vi "Simple Endpoint Control.vi"(3 "error in":errorcluster, 4 "Side":T1=enum."right", 5 "Position":T2={"Theta"=-42.91139240506329, "r"=17.78481012658228, "wrist"=-20.886075949367083, "Z"=0.25316455696202533} {"Z" scale=-10.0..10.0; "wrist" scale=-90.0..90.0; "r" scale=10.0..25.0; "Theta" scale=-90.0..90.0}) -> (0 "error out":errorcluster)   [LabVIEW 2010]
uses:
  <userlib>/ROSforLV_0.1/ROS/Code/SubVIs/BaxterArmsSmall.ctl
  <userlib>/ROSforLV_0.1/ROS/Code/SubVIs/BaxterSide.ctl
panel:
  out "g":dbl=49.666540029773564
  out "x":dbl=17.786611918279583
  out "p":dbl=0.8155432028971262
  out "a":dbl=54.75975470538772
  in  "Start":T3={"Elbow 0"=0.0, "Elbow 1"=55.8123726628928, "Shoulder 0"=0.0, "Shoulder 1"=-28.952431226064945, "Wrist 0"=0.0, "Wrist 1"=63.14005856317215, "Wrist 2"=0.0}
  out "Arm Angles (degrees)":T3={"Elbow 0"=0.0, "Elbow 1"=104.42629473516128, "Shoulder 0"=-42.91139240506329, "Shoulder 1"=-55.575297908284846, "Wrist 0"=0.0, "Wrist 1"=41.14900317312356, "Wrist 2"=-20.886075949367083}
  in  "d 4":dbl=10.0
  in  "d 3":dbl=15.0
  in  "d 2":dbl=14.0
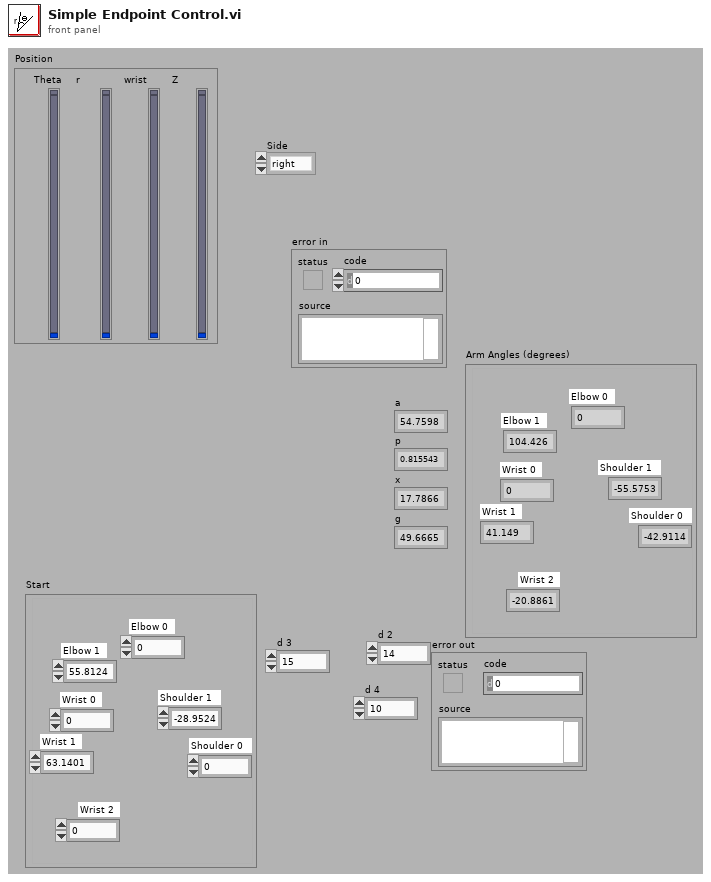
[diagram p1: front panel]
types:
  T1 = typedef "BaxterSide.ctl" = enum16{"left", "right"}
  T2 = cluster{"Theta":dbl, "r":dbl, "wrist":dbl, "Z":dbl}
  T3 = typedef "BaxterArmsSmall.ctl" = cluster{"Elbow 0":dbl, "Elbow 1":dbl, "Shoulder 0":dbl, "Shoulder 1":dbl, "Wrist 0":dbl, "Wrist 1":dbl, "Wrist 2":dbl}
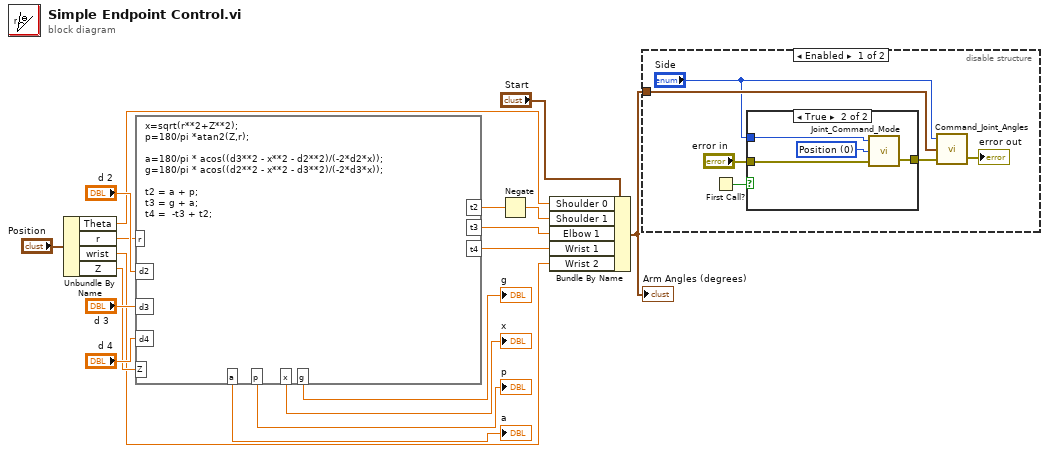
[diagram p0: block diagram]
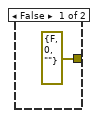
[diagram p2: hidden frame]
diagram:
  n1 = Unbundle By Name("Position") -> ("Theta"=w4:dbl, "r"=w3:dbl, "wrist"=w1:dbl, "Z"=w2:dbl)
  n2 = formula code="x=sqrt(r**2+Z**2);\np=180/pi *atan2(Z,r);\n\na=180/pi * acos((d3**2 - x**2 - d2**2)/(-2*d2*x));\ng=180/pi * acos((d2**2 - x**2 - d3**2)/(-2*d3*x));\n\nt2 = a + p;\nt3 = g + a;\nt4 =  -t3 + t2;"("r"=w3, "d2"="d 2", "d3"="d 3", "d4"="d 4", "Z"=w2) -> ("t2"=w13:dbl, "t3"=w12:dbl, "t4"=w11:dbl, "a"=→"a":dbl, "p"=→"p":dbl, "x"=→"x":dbl, "g"=→"g":dbl)
  n3 = Negate(x=w13) -> (-x=w6:dbl)
  n4 = Bundle By Name(cluster="Start", "Shoulder 0"=w4, "Shoulder 1"=w6, "Elbow 1"=w12, "Wrist 1"=w11, "Wrist 2"=w1) -> (w17:T3)
  "Arm Angles (degrees)" <- w17
  n5 = disable-structure shown="Enabled" {
    disable-tunnel: w17 -> [w24 _]
    frame Enabled {
      n6 = First Call?() -> (First Call?: T/F=w22:bool)
      n7 = case shown="True" w22 {
        tunnel: [errorcluster {"status"=FALSE, "code"=0, "source"=""} ("error out") w28] -> w23
        tunnel: "Side" -> [_ w27]
        tunnel: "error in" -> [_ w26]
        frame False {
        }
        frame True {
          w29 = u8 0 items=["Position", "Velocity", "Effort"] ("Mode")
          n8 = call <userlib>:"Joint_Command_Mode.vi"("Side"=w27, "Mode"=w29, "error in"=w26) -> ("error out"=w28:errorcluster)  [unwired: 3 in]
        }
      }
      n9 = call <userlib>:"Command_Joint_Angles.vi"("Side"="Side", "Arm Angles (degrees)"=w24, "error in"=w23) -> ("error out"=→"error out":errorcluster)  [unwired: 3 in]
    }
    frame Disabled {
    }
  }
